vi "PH_Sixpack.SetVMinVStart.vi"(0 "i ref in":refnum<vi>, 1 "axis":i32=-1, 4 "Device Error in":errorcluster, 5 "error in":errorcluster) -> (14 "i ref out":refnum<vi>, 16 "ok?":bool, 18 "Device Error out":errorcluster, 19 "error out":errorcluster)   [LabVIEW 2014, in "PH_Sixpack.lvlib"]
doc: "This VI acts on the hardware."
uses:
  PH_Sixpack.lvlib
  instr.lib/Sixpack/Sixpack - Driver.lvlib
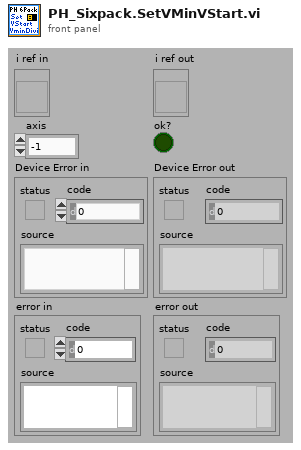
[diagram p1: front panel]
types:
  T1 = typedef "PH_Sixpack.lvlib/PH_Sixpack.Axis Cluster.ctl" = cluster{"Config":T2, "To set?":cluster{"VmaxAmax":bool, "I max":bool, "VStartVminDivi":bool, "Ref Search Parameter":bool, "Stopswitch Limits":bool, "Axis Parameter":bool, "I Control":bool}}
  T2 = typedef "PH_Sixpack.lvlib/PH_Sixpack.Axis Configuration.ctl" = cluster{"VmaxAmax":T3, "I max (50%)":T4, "VStartVminDivi":T5, "Ref Search Parameter":T6, "Stopswitch Limits":T7, "Axis Parameter":T8, "I Control":T11}
  T3 = typedef "Sixpack - Driver.lvlib/VmaxAmax.ctl" = cluster{"VMax(511)":u16, "AMax(128)":u16}
  T4 = typedef "Sixpack - Driver.lvlib/PeakCurrent.ctl" = dbl
  T5 = typedef "Sixpack - Driver.lvlib/VStartVmin.ctl" = cluster{"VStart(5)":u16, "Vmin(4)":u16, "Div i (2)":enum8{"0", "1", "2", "3"}}
  T6 = typedef "Sixpack - Driver.lvlib/Ref Search Parameter.ctl" = cluster{"VRefMax(100)":u16, "DebouncingTime (22ms)":u8}
  T7 = typedef "Sixpack - Driver.lvlib/Stopswitch Limits.ctl" = cluster{"MinLeft(0)":u16, "MaxRight(1023)":u16}
  T8 = typedef "Sixpack - Driver.lvlib/Motor Parameter.ctl" = cluster{"Poslimit (6400)":u32, "P5 Bits":T9, "P6 Bits":T10}
  T9 = typedef "Sixpack - Driver.lvlib/MotorParameter_P5.ctl" = cluster{"MT_PI":bool, "MT_ROTARY":bool, "MT_AUTONULLCMD":bool, "MT_TESTNULL":bool, "MT_NULLLEFT":bool, "MT_NULLCENTRE":bool, "MT_STOPNULL":bool, "MT_FILTERSWITCH":bool}
  T10 = typedef "Sixpack - Driver.lvlib/MotorParameter_P6.ctl" = cluster{"MT_OPTIMIZEWAY":bool, "MT_FASTREF":bool, "MT_MECHREF":bool, "MT_DELAYTESTNULL":bool, "MT_STOPSOFT":bool, "MT_STOPNOREF":bool, "MT_NULLPOSITIVE":bool, "MUT_STOPFULSTEPS":bool}
  T11 = typedef "Sixpack - Driver.lvlib/Current Control.ctl" = cluster{"PowerDownDelay (500)":u16, "PowerDown (0%)":T12, "Standing (50%)":T12, "Running (75%)":T12, "Accelerating (100%)":T12}
  T12 = typedef "Sixpack - Driver.lvlib/Current.ctl" = enum8{"100%", "75%", "50%", "38%", "25%", "19%", "13%", "9%", "0%"}
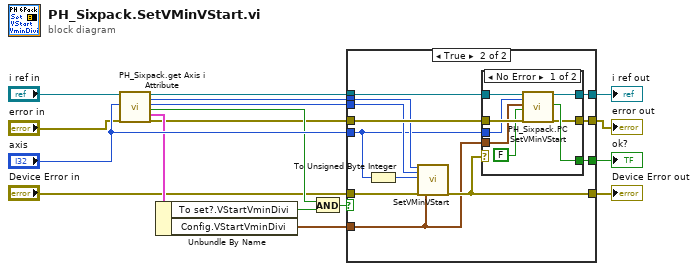
[diagram p0: block diagram]
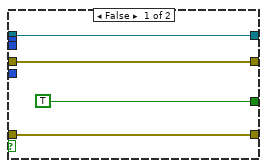
[diagram p2: hidden frame]
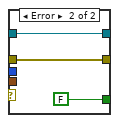
[diagram p3: hidden frame]
diagram:
  n1 = call "PH_Sixpack.get Axis i Attribute.vi"("VI in"="i ref in", "Axis"="axis", "error in"="error in") -> ("VI out"=w14:refnum<vi>, "HANDLE"=w7:i32, "SixPack ID(0)"=w6:u16, "Axis found?"=w11:bool, "Axis Attributes"=w12:T1, "error out"=w4:errorcluster)  [unwired: 10 in, 1 out]
  n2 = Unbundle By Name(w12) -> ("To set?.VStartVminDivi"=w1:bool, "Config.VStartVminDivi"=w2:T5)
  n3 = And(x=w11, y=w1) -> (x .and. y?=w8:bool)
  n4 = case shown="True" w8 {
    tunnel: w4 -> [w19 w33]
    tunnel: [w19 w32] -> w16
    tunnel: [w20 w31] -> w15
    tunnel: w14 -> [w20 w30]
    tunnel: "axis" -> [_ w25]
    tunnel: [w21 w29] -> w10
    tunnel: "Device Error in" -> [w21 w28]
    tunnel: w2 -> [_ w22]
    tunnel: w7 -> [_ w27]
    tunnel: w6 -> [_ w26]
    tunnel: [TRUE w23] -> w3
    frame False {
    }
    frame True {
      n5 = To Unsigned Byte Integer(number=w25) -> (unsigned 8bit integer=w24:u8)
      n6 = call "SetVMinVStart.vi"("handle in"=w27, "UnitAddress(0)"=w26, "MotNr(0)"=w24, "error in"=w28, "VminVStart"=w22) -> ("error out"=w29:errorcluster)  [unwired: 13 in, 1 out]
      n7 = case shown="No Error" w29 {
        tunnel: w33 -> [w41 w43]
        tunnel: [w37 w43] -> w32
        tunnel: [w38 w44] -> w31
        tunnel: w30 -> [w40 w44]
        tunnel: w25 -> [w36 _]
        tunnel: [w39 FALSE] -> w23
        tunnel: w22 -> [w35 _]
        frame No Error {
          n8 = call "PH_Sixpack.PC SetVMinVStart.vi"("i ref in"=w40, "axis"=w36, "VStartVminDivi"=w35, "To Set?"=FALSE, "error in (no error)"=w41) -> ("i ref out"=w38:refnum<vi>, "ok?"=w39:bool, "error out"=w37:errorcluster)  [unwired: 12 in]
        }
        frame Error {
        }
      }
    }
  }
  "error out" <- w16
  "i ref out" <- w15
  "Device Error out" <- w10
  "ok?" <- w3
